vi "Validate Device Data to Search.vi"(8 "error in (no error)":errorcluster) -> (0 "error out":errorcluster, 3 "Valid Device?":bool)   [LabVIEW 2024, in "User Interface.lvlib"]
doc: "Validates whether IP address, username and hostname are valid fields.\n-No blank spaces between characters\n-Valid IP address syntax\n\nIn case user enters IP address and hostname the VI will validate both fields are OK, otherwise, the VI will validate at least one between IP address or hostname will be OK."
uses:
  User Interface.lvlib
  <vilib>/Utility/error.llb/Trim Whitespace One-Sided.vi
  Support/General Type Defs/Global Data.vi
  Support/General Type Defs/General Type Defs.lvlib
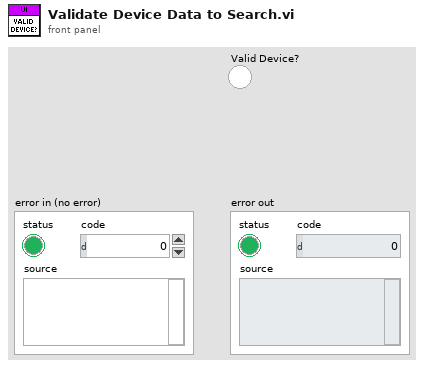
[diagram p1: front panel]
types:
  T1 = typedef "General Type Defs.lvlib/Device Data.ctl" = cluster{"OS":T2, "User":string, "Password":string, "Hostname":string, "IP Address":string}
  T2 = typedef "General Type Defs.lvlib/Device OS.ctl" = enum16{"Windows", "Linux"}
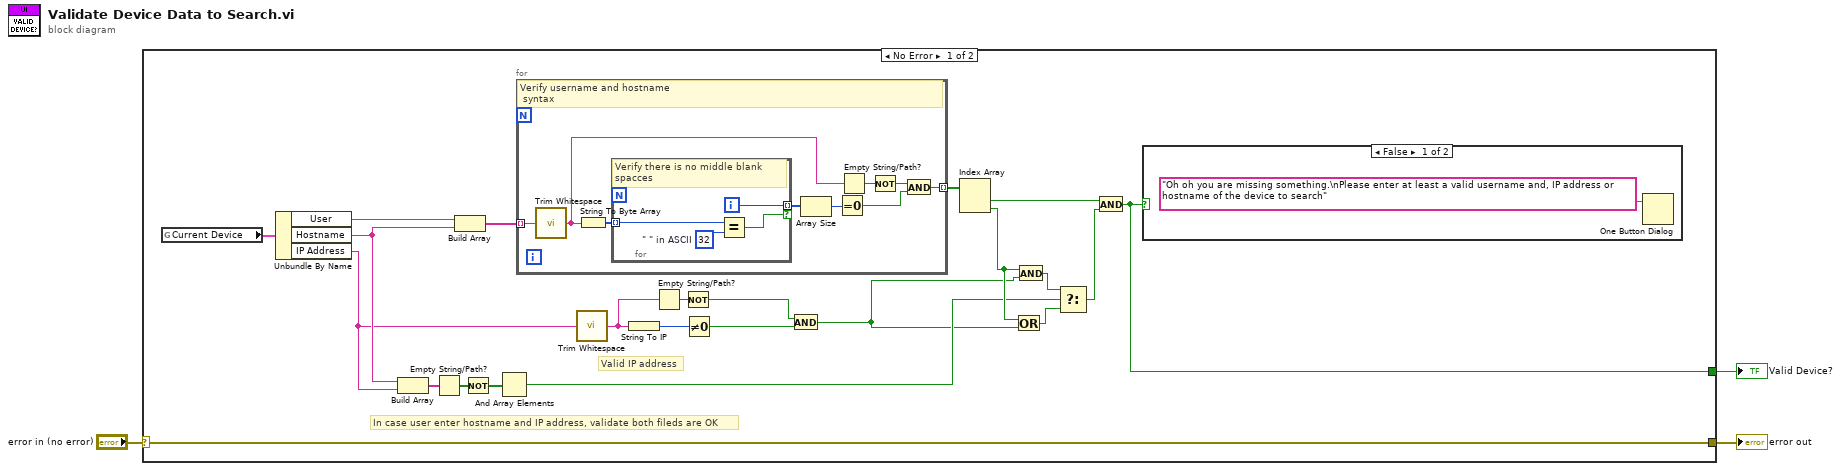
[diagram p0: block diagram]
diagram:
  n1 = case shown="No Error" "error in (no error)" {
    selector: "error in (no error)" -> [w26 w41]
    tunnel: [w26 w41] -> w3
    tunnel: [w4 _] -> w1
    frame No Error {
      # "Valid IP address"
      # "In case user enter hostname and IP address, validate both fileds are OK"
      n2 = global read "Global Data.vi" "Current Device"() -> (w5:T1)
      n3 = Unbundle By Name(w5) -> ("User"=w25:string, "Hostname"=w18:string, "IP Address"=w12:string)
      n4 = Build Array(w18, w12) -> (w17:string[])
      n5 = Empty String/Path?(string/path=w17) -> (empty?=w16:bool[])
      n6 = Build Array(w25, w18) -> (w24:string[])
      n7 = Not(x=w16) -> (.not. x?=w15:bool[])
      n8 = And Array Elements(Boolean array=w15) -> (logical AND=w14:bool)
      n9 = for {
        tunnel: [w27] -> w23 mode=indexing
        tunnel: w24 -> [w32] mode=indexing
        # "Verify username and hostname\n syntax"
        n10 = call <vilib>:"Trim Whitespace.vi"("string"=w32) -> ("trimmed string"=w29:string)  [unwired: 1 in]
        n11 = String To Byte Array(string=w29) -> (unsigned byte array=w35:u8[])
        n12 = for {
          tunnel: w35 -> [w39] mode=indexing
          tunnel: [w37] -> w34 mode=indexing if=w36
          i -> [w37]
          w38 = u8 32  # " " in ASCII
          # "Verify there is no middle blank\nspacces"
          n13 = Equal?(x=w39, y=w38) -> (x = y?=w36:bool)
        }
        n14 = Array Size(array=w34) -> (size(s)=w33:i32)
        n15 = Equal To 0?(x=w33) -> (x = 0?=w30:bool)
        n16 = Empty String/Path?(string/path=w29) -> (empty?=w31:bool)
        n17 = Not(x=w31) -> (.not. x?=w28:bool)
        n18 = And(x=w28, y=w30) -> (x .and. y?=w27:bool)
      }
      n19 = call <vilib>:"Trim Whitespace.vi"("string"=w12) -> ("trimmed string"=w8:string)  [unwired: 1 in]
      n20 = String To IP(1:w8) -> (0:w11:u32)
      n21 = Empty String/Path?(string/path=w8) -> (empty?=w9:bool)
      n22 = Not(x=w9) -> (.not. x?=w6:bool)
      n23 = Not Equal To 0?(x=w11) -> (x != 0?=w10:bool)
      n24 = And(x=w6, y=w10) -> (x .and. y?=w7:bool)
      n25 = Index Array(array=w23) -> (element #1=w22:bool, element #2=w19:bool)  [unwired: 2 in]
      n26 = Or(x=w19, y=w7) -> (x .or. y?=w21:bool)
      n27 = And(x=w19, y=w7) -> (x .and. y?=w20:bool)
      n28 = Select(t=w20, s=w14, f=w21) -> (s? t:f=w13:bool)
      n29 = And(x=w22, y=w13) -> (x .and. y?=w4:bool)
      n30 = case shown="False" w4 {
        frame False {
          n31 = One Button Dialog(message="Oh oh you are missing something.\nPlease enter at least a valid username and, IP address or hostname of the device to search") -> ()  [unwired: 1 in, 1 out]
        }
        frame True {
        }
      }
    }
    frame Error {
    }
  }
  "Valid Device?" <- w1
  "error out" <- w3
